vi "(SubVI) Fixed-Window Average Filters_YCC.vi"(5 "Avg points":i32, 7 "Signal":dbl[](array[numeric])) -> (3 "Filtered Signal":dbl[](array[numeric]))   [LabVIEW 2014]
uses:
  <vilib>/Analysis/baseanly.llb/Mean (DBL).vi
  <vilib>/Analysis/NI_AALBase.lvlib
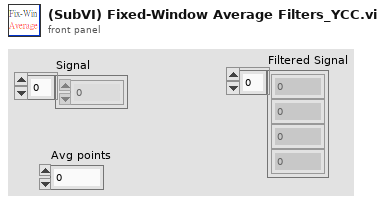
[diagram p1: front panel]
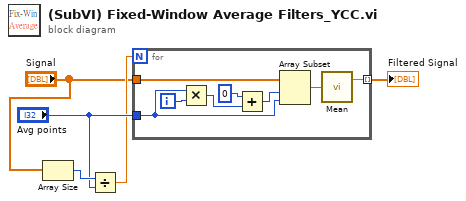
[diagram p0: block diagram]
diagram:
  n1 = Array Size(array="Signal") -> (size(s)=w4:i32)
  n2 = Divide(x=w4, y="Avg points") -> (x/y=w2:dbl)
  n3 = for {
    N: w2 -> [_]
    tunnel: "Signal" -> [w13]
    tunnel: "Avg points" -> [w9]
    tunnel: [w11] -> w5 mode=indexing
    i -> [w10]
    n4 = Multiply(x=w9, y=w10) -> (x*y=w8:i32)
    n5 = Add(x=0 ("index"), y=w8) -> (x+y=w6:i32)
    n6 = Array Subset(array=w13, index=w6, length=w9) -> (w12:dbl[])
    n7 = call-poly <vilib>:"Mean.vi"("X"=w12) -> ("mean"=w11:dbl)  [unwired: 1 out]
  }
  "Filtered Signal" <- w5
